vi "filterFlatData.vi"(8 "Data with flat data 2":T1(array[cluster]), 11 "Data with flat data":T1(array[cluster])) -> (0 "Data without flat data 2":cluster{"name":string, "type desc":i16[]}[](array[cluster]), 3 "Data without flat data":cluster{"name":string, "type desc":i16[]}[](array[cluster]))   [LabVIEW 2010]
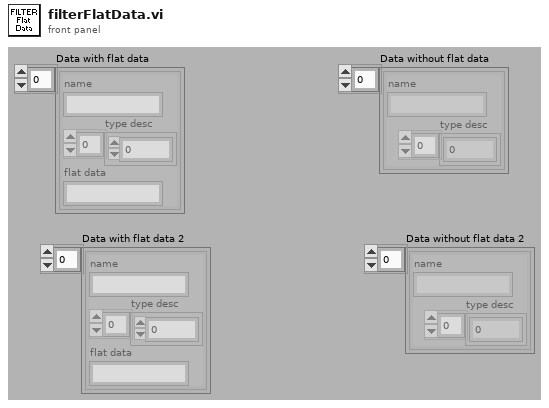
[diagram p1: front panel]
types:
  T1 = cluster{"name":string, "type desc":i16[], "flat data":string}[]
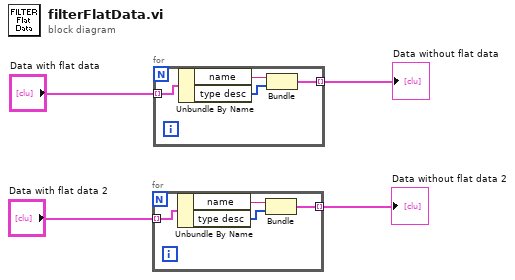
[diagram p0: block diagram]
diagram:
  n1 = for {
    tunnel: "Data with flat data 2" -> [w8] mode=indexing
    tunnel: [w5] -> w1 mode=indexing
    n2 = Unbundle By Name(w8) -> ("name"=w7:string, "type desc"=w6:i16[])
    n3 = Bundle("name"=w7, "type desc"=w6) -> (w5:cluster{"name":string, "type desc":i16[]})  [unwired: 1 out]
  }
  "Data without flat data 2" <- w1
  n4 = for {
    tunnel: "Data with flat data" -> [w12] mode=indexing
    tunnel: [w9] -> w3 mode=indexing
    n5 = Unbundle By Name(w12) -> ("name"=w11:string, "type desc"=w10:i16[])
    n6 = Bundle("name"=w11, "type desc"=w10) -> (w9:cluster{"name":string, "type desc":i16[]})  [unwired: 1 out]
  }
  "Data without flat data" <- w3
